vi "Self Test.vi"(8 "error in (no error)":errorcluster, 11 "VISA resource name":refnum<visa-resource-name>) -> (0 "error out":errorcluster, 1 "Self-Test Response":string, 2 "self-test error":bool, 3 "VISA resource name out":refnum<visa-resource-name>)   [LabVIEW 2020, in "Agilent 6XXX Series.lvlib"]
doc: "This VI causes the instrument to perform a self-test and returns the results. A boolean indicates if the instrument passed self-test, and string contains the instruments reponse."
uses:
  <instrlib>/Agilent 6XXX Series/Agilent 6XXX Series.lvlib
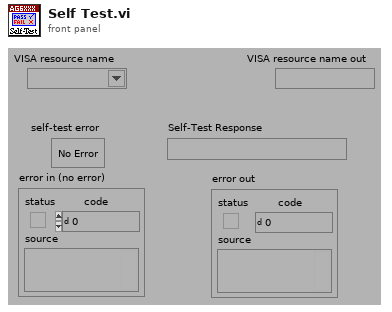
[diagram p1: front panel]
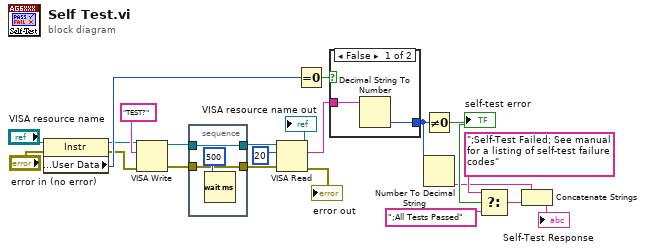
[diagram p0: block diagram]
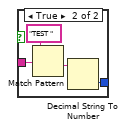
[diagram p2: hidden frame]
diagram:
  n1 = property class="Instr"(reference="VISA resource name", error in="error in (no error)") -> (reference out=w2:refnum<visa-resource-name>, error out=w1:errorcluster, "General Settings:User Data"=w3:u32)
  n2 = VISA Write(VISA resource name=w2, write buffer="TEST?" ("self-test command"), error in (no error)=w1) -> (VISA resource name out=w17:refnum<visa-resource-name>, error out=w18:errorcluster)  [unwired: 1 out]
  n3 = stacked-sequence {
    tunnel: w18 -> [w24]
    tunnel: w17 -> [w23]
    tunnel: [w24] -> w16
    tunnel: [w23] -> w15
    frame #0 {
      n4 = Wait (ms)(milliseconds to wait=u32 500) -> ()  [unwired: 1 out]
    }
  }
  n5 = VISA Read(VISA resource name=w15, byte count=u32 20, error in (no error)=w16) -> (VISA resource name out=→"VISA resource name out":refnum<visa-resource-name>, read buffer=w6:string, error out=→"error out":errorcluster)  [unwired: 1 out]
  n6 = Equal To 0?(x=w3) -> (x = 0?=w8:bool)
  n7 = case shown="False" w8 {
    tunnel: [w26 w29] -> w5
    tunnel: w6 -> [w27 w28]
    frame False {
      n8 = Decimal String To Number(string=w27) -> (number=w26:i32)  [unwired: 2 in, 1 out]
    }
    frame True {
      n9 = Match Pattern(string=w28, regular expression="TEST ") -> (after substring=w30:string)  [unwired: 1 in, 3 out]
      n10 = Decimal String To Number(string=w30) -> (number=w29:i32)  [unwired: 2 in, 1 out]
    }
  }
  n11 = Not Equal To 0?(x=w5) -> (x != 0?=w7:bool)
  "self-test error" <- w7
  n12 = Number To Decimal String(number=w5) -> (decimal integer string=w4:string)  [unwired: 1 in]
  n13 = Select(t=";Self-Test Failed; See manual for a listing of self-test failure codes", s=w7, f=";All Tests Passed") -> (s? t:f=w12:string)
  n14 = Concatenate Strings(w4, w12) -> (→"Self-Test Response":string)
